vi "IMAQ FPGA Wait for Image Transfer Complete U8.vi"(5 "Wait Timeout (ms)":i32=5000, 7 "DMA FIFO Depth in Elements":u32, 8 "error in (no error)":errorcluster, 9 "DMA FIFO Reference In":refnum<k20>, 10 "Source FIFO Status Indicator Name":string, 11 "FPGA VI Reference In":refnum<k20>) -> (0 "error out":errorcluster, 1 "DMA FIFO Reference Out":refnum<k20>)   [LabVIEW 2020, in "NI_VDM_FPGA_Basics.lvlib"]
doc: "Waits for the transfer of image data from the host processor to the target FPGA via a DMA FIFO to complete or for the specified timeout to expire before returning. The transfer is deemed complete when the host-side buffer of the DMA FIFO is empty and the DMA FIFO on the FPGA is empty as well. To ensure that none of the image data will be lost, call this VI after the last call to the IMAQ FPGA Image Transfer to Target VI and prior to calling the Close FPGA VI Reference function on the DMA FIFO Reference."
uses:
  <vilib>/visionFPGA/NI_VDM_FPGA_Basics.lvlib
  <vilib>/visionFPGA/Controls/IMAQ FPGA Source FIFO Status.ctl
  <vilib>/NI/LVFPGA Adv Session Resources/OpenByNameSubVI.vi
  <vilib>/rvi/errors/niLvFpgaAdjustHostInterfaceError.vi
  <vilib>/rvi/interface/common/dynamic/niFpgaEscapeDelimiterAndNull.vi
  <vilib>/FPGAPlugInAG/Dynamic/niLvFpga_Close_Dynamic.vi
  <vilib>/rvi/interface/nirviMethod/nirviMethod.xnode
  <vilib>/NI/LVFPGA Adv Session Resources/OpenByName.xnode
  <vilib>/rvi/interface/nirviReadWriteControl/nirviReadWriteControl.xnode
  <vilib>/rvi/interface/nirviCloseFPGA/nirviCloseFPGA.xnode
  <vilib>/NI/LVFPGA Adv Session Resources/LVFPGAAdvSessionResources.lvlib
  NiFpgaLv.dll
  <vilib>/rvi/interface/Simulation/niFpgaSimulationCallBeginRW.vi
  <vilib>/FPGAPlugInAG/Dynamic/niLvFpga_WriteFifo_Dynamic.vi
  <vilib>/rvi/errors/niLvFpgaMergeErrorWithErrorCode.vi
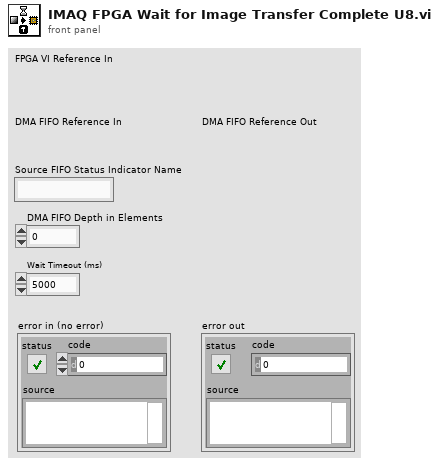
[diagram p1: front panel]
types:
  T1 = typedef "IMAQ FPGA Source FIFO Status.ctl" = cluster{"Number of Elements to Read":u32}
  T2 = enum16{"Register", "Host To Target FIFO", "Target To Host FIFO"}
  T3 = cluster{"Name":string, "Depth":u32, "Write? (Deprecated:Use Implementation)":bool, "Physical Channel":u32, "Base Address":u32, "Data Width":u32, "Data Type":enum32{"Boolean", "I8", "I16", "I32", "I64", "U8", "U16", "U32", "U64", "FXP", "CustomControl", "SGL"}, "FXP Properties":variant, "Write Window Address":u32, "Implementation":enum16{"niFpgaTargetToHost", "niFpgaHostToTarget", "niFpgaPeerToPeerWriter", "niFpgaPeerToPeerReader", "niCoreTargetToHost", "niCoreHostToTarget"}, "Control Set":u32}[]
  T4 = cluster{"Name":string, "type":variant, "indicator?":bool}[]
  T5 = typedef "LVFPGAAdvSessionResources.lvlib/ResourceInfo.ctl" = cluster{"Resource name":string, "Data type":variant, "Resource type":enum16{"Register", "Host To Target FIFO", "Target To Host FIFO"}}
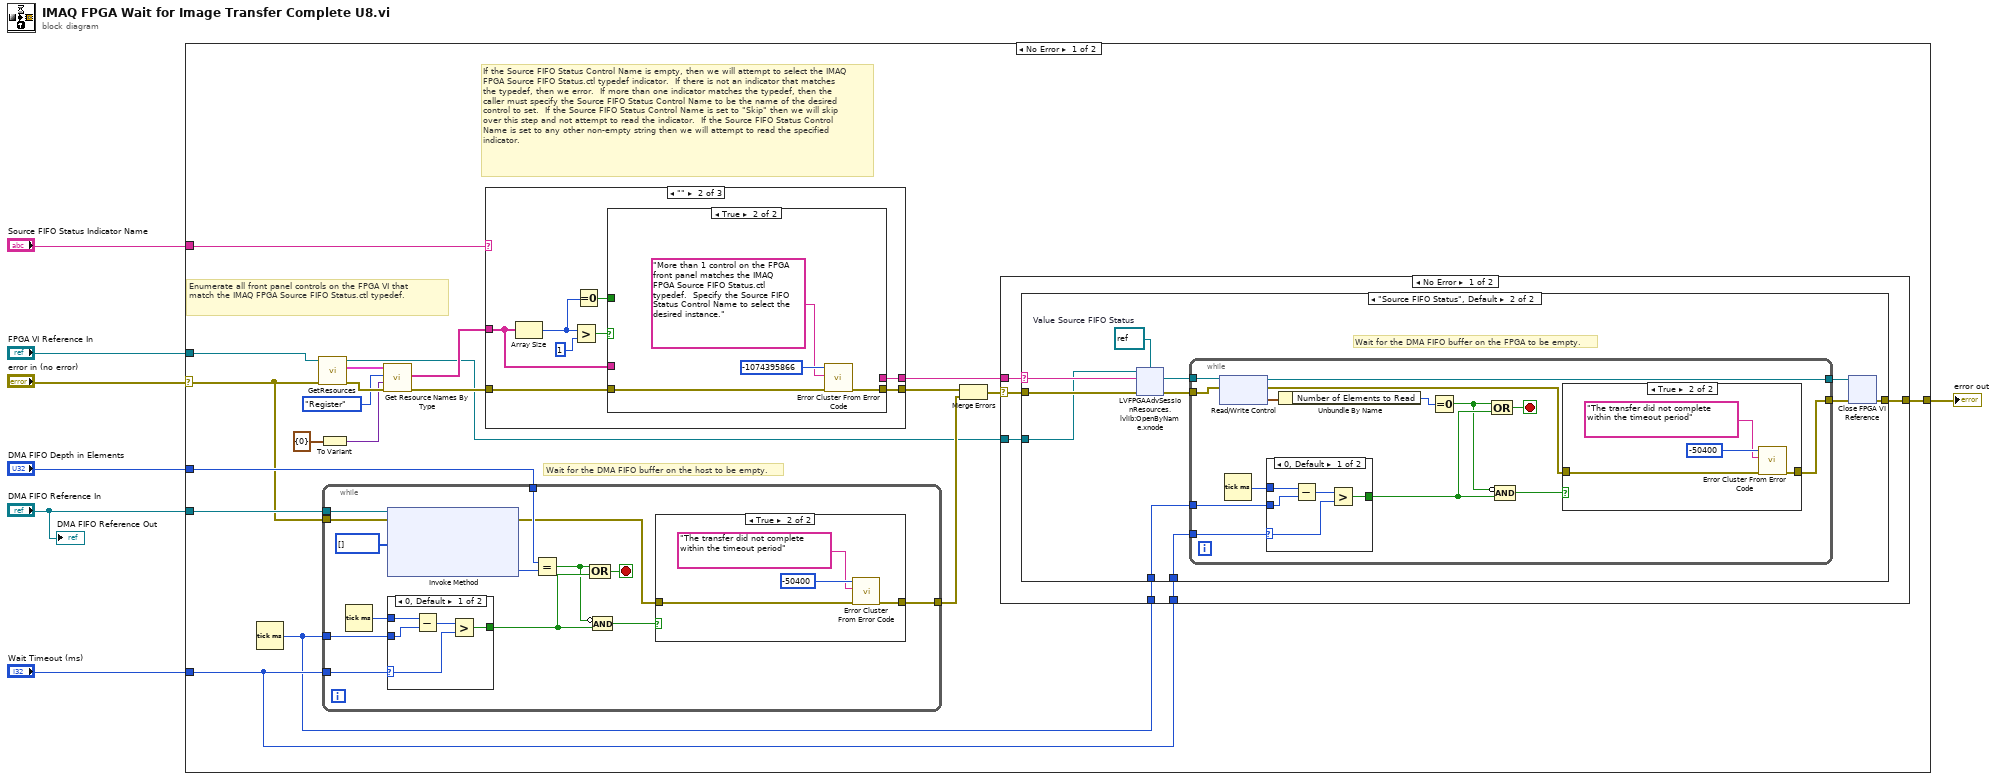
[diagram p0: block diagram]
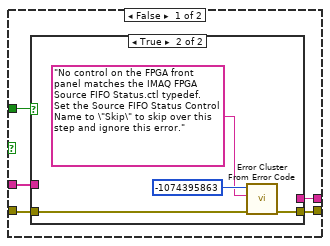
[diagram p7: hidden frame]
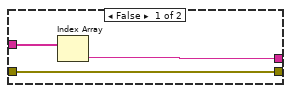
[diagram p8: hidden frame]
diagram:
  n1 = case shown="No Error" "error in (no error)" {
    selector: "error in (no error)" -> [w8 w135]
    tunnel: "DMA FIFO Depth in Elements" -> [w27 _]
    tunnel: "FPGA VI Reference In" -> [w23 _]
    tunnel: "Source FIFO Status Indicator Name" -> [w21 _]
    tunnel: "Wait Timeout (ms)" -> [w13 _]
    tunnel: [w11 w135] -> w3
    tunnel: "DMA FIFO Reference In" -> [w10 _]
    frame No Error {
      # "Wait for the DMA FIFO buffer on the host to be empty."
      # "If the Source FIFO Status Control Name is empty, then we will attempt to select the IMAQ FPGA Source FIFO Status.ctl typedef indicator.  If there is not an indicator that matches the typedef, then we error.  If more than one indicator matches the typedef, then the caller must specify the Source FIFO Status Control Name to be the name of the desired control to set.  If the Source FIFO Status Control Name is set to \"Skip\" then we will skip over this step and not attempt to read the indicator.  If the Source FIFO Status Control Name is set to any other non-empty string then we will attempt to read the specified indicator."
      # "Enumerate all front panel controls on the FPGA VI that match the IMAQ FPGA Source FIFO Status.ctl typedef."
      n2 = Tick Count (ms)() -> (millisecond timer value=w12:u32)
      n3 = call <vilib>:"GetResources.vi"("error in (no error)"=w8, "FPGA VI Reference in"=w23) -> ("error out"=w26:errorcluster, "Resource info out"=w24:T5[], "FPGA VI Reference out"=w14:refnum<k20>)  [unwired: 7 in]
      n4 = To Variant(anything=T1 {"Number of Elements to Read"=0} ("Source FIFO Status")) -> (Variant=w19:variant)
      n5 = while {
        tunnel: w10 -> [w124]
        tunnel: w27 -> [w122]
        tunnel: w8 -> [w121]
        tunnel: w12 -> [w118]
        tunnel: w13 -> [w119]
        tunnel: [w111] -> w16
        stop <- w116 stop-if-true
        n6 = Tick Count (ms)() -> (millisecond timer value=w117:u32)
        n7 = case shown="0, Default" w119 {
          selector: w119 -> [w131 _]
          tunnel: w118 -> [w133 _]
          tunnel: w117 -> [w134 _]
          tunnel: [w130 _] -> w115
          frame 0, Default {
            n8 = Subtract(x=w134, y=w133) -> (x-y=w132:u32)
            n9 = Greater?(x=w132, y=w131) -> (0:w130:bool)
          }
          frame -1 {
          }
        }
        n10 = xnode "Invoke Method"("FPGA VI Reference In"=w124, "error in"=w121, "Data"=u8[] []) -> ("error out"=w112:errorcluster, "Empty Elements Remaining"=w123:u32)  [unwired: 1 in, 1 out]
        n11 = Equal?(x=w122, y=w123) -> (x = y?=w114:bool)
        n12 = Compound Arithmetic op=OR(w114, w115) -> (w116:bool)
        n13 = Compound Arithmetic op=AND(invert w114, w115) -> (w113:bool)
        n14 = case shown="True" w113 {
          tunnel: w112 -> [w125 w129]
          tunnel: [w125 w128] -> w111
          frame False {
          }
          frame True {
            n15 = call <vilib>:"Error Cluster From Error Code.vi"("error in (no error)"=w129, "error message (\"\")"="The transfer did not complete within the timeout period" ("error message (\"\")"), "error code (0)"=-50400) -> ("error out"=w128:errorcluster)  [unwired: 6 in]
          }
        }
      }
      n16 = call <vilib>:"Get Resource Names By Type.vi"("error in (no error)"=w26, "Data Type"=w19, "Resource Type"=T2."Register", "Resource Info In"=w24) -> ("error out"=w20:errorcluster, "Resource Names"=w22:string[])  [unwired: 5 in, 1 out]
      n17 = case shown="\"\"" w21 {
        selector: w21 -> [w84 _ _]
        tunnel: w20 -> [w85 w92 w110]
        tunnel: [w85 w91 w110] -> w17
        tunnel: [w84 w90 _] -> w18
        tunnel: w22 -> [_ w88 _]
        frame "Anything Else", Default {
        }
        frame "" {
          n18 = Array Size(array=w88) -> (size(s)=w86:i32)
          n19 = Greater?(x=w86, y=1 ("x")) -> (0:w93:bool)
          n20 = Equal To 0?(x=w86) -> (x = 0?=w87:bool)
          n21 = case shown="True" w93 {
            tunnel: w88 -> [w98 _]
            tunnel: [w97 _] -> w90
            tunnel: [w95 w107] -> w91
            tunnel: w92 -> [w96 w106]
            tunnel: w87 -> [w94 _]
            frame False {
              n22 = case shown="True" w94 {
                tunnel: w98 -> [w101 _]
                tunnel: [w100 _] -> w97
                tunnel: w96 -> [w99 w103]
                tunnel: [w99 w102] -> w95
                frame False {
                  n23 = Index Array(array=w101) -> (element=w100:string)  [unwired: 1 in]
                }
                frame True {
                  n24 = call <vilib>:"Error Cluster From Error Code.vi"("error in (no error)"=w103, "error message (\"\")"="No control on the FPGA front panel matches the IMAQ FPGA Source FIFO Status.ctl typedef.  Set the Source FIFO Status Control Name to \"Skip\" to skip over this step and ignore this error." ("error message (\"\")"), "error code (0)"=-1074395863) -> ("error out"=w102:errorcluster)  [unwired: 6 in]
                }
              }
            }
            frame True {
              n25 = call <vilib>:"Error Cluster From Error Code.vi"("error in (no error)"=w106, "error message (\"\")"="More than 1 control on the FPGA front panel matches the IMAQ FPGA Source FIFO Status.ctl typedef.  Specify the Source FIFO Status Control Name to select the desired instance." ("error message (\"\")"), "error code (0)"=-1074395866) -> ("error out"=w107:errorcluster)  [unwired: 6 in]
            }
          }
        }
        frame "Skip" {
        }
      }
      n26 = Merge Errors(w17, w16) -> (w15:errorcluster)
      n27 = case shown="No Error" w15 {
        selector: w15 -> [w32 w83]
        tunnel: w18 -> [w33 _]
        tunnel: w14 -> [w31 _]
        tunnel: w13 -> [w30 _]
        tunnel: w12 -> [w29 _]
        tunnel: [w28 w83] -> w11
        frame No Error {
          n28 = case shown="\"Source FIFO Status\", Default" w33 {
            selector: w33 -> [_ w44]
            tunnel: w32 -> [w34 w43]
            tunnel: w31 -> [_ w42]
            tunnel: w30 -> [_ w37]
            tunnel: w29 -> [_ w36]
            tunnel: [w34 w35] -> w28
            frame "" {
            }
            frame "Source FIFO Status", Default {
              w45 = refnum<k20> refnum  # Value Source FIFO Status
              # "Wait for the DMA FIFO buffer on the FPGA to be empty."
              n29 = xnode "LVFPGAAdvSessionResources.lvlib:OpenByName.xnode"("FPGA VI Reference in"=w42, "Resource name in"=w44, "Single resource reference type in"=w45, "Error in"=w43) -> ("Single resource reference out"=w38:refnum<k20>, "Error out"=w41:errorcluster)  [unwired: 1 out]
              n30 = while {
                tunnel: w38 -> [w72]
                tunnel: w41 -> [w71]
                tunnel: [w59] -> w40
                tunnel: [w70] -> w39
                tunnel: w37 -> [w66]
                tunnel: w36 -> [w65]
                stop <- w64 stop-if-true
                n31 = xnode "Read/Write Control"("FPGA VI Reference In"=w72, "error in"=w71) -> ("FPGA VI Reference Out"=w70:refnum<k20>, "error out"=w61:errorcluster, "Value"=w68:cluster{"Number of Elements to Read":u32})
                n32 = Tick Count (ms)() -> (millisecond timer value=w67:u32)
                n33 = case shown="0, Default" w66 {
                  selector: w66 -> [w79 _]
                  tunnel: w65 -> [w81 _]
                  tunnel: w67 -> [w82 _]
                  tunnel: [w78 _] -> w63
                  frame 0, Default {
                    n34 = Subtract(x=w82, y=w81) -> (x-y=w80:u32)
                    n35 = Greater?(x=w80, y=w79) -> (0:w78:bool)
                  }
                  frame -1 {
                  }
                }
                n36 = Unbundle By Name(w68) -> ("Number of Elements to Read"=w69:u32)
                n37 = Equal To 0?(x=w69) -> (x = 0?=w62:bool)
                n38 = Compound Arithmetic op=OR(w62, w63) -> (w64:bool)
                n39 = Compound Arithmetic op=AND(invert w62, w63) -> (w60:bool)
                n40 = case shown="True" w60 {
                  tunnel: w61 -> [w73 w77]
                  tunnel: [w73 w76] -> w59
                  frame False {
                  }
                  frame True {
                    n41 = call <vilib>:"Error Cluster From Error Code.vi"("error in (no error)"=w77, "error message (\"\")"="The transfer did not complete within the timeout period" ("error message (\"\")"), "error code (0)"=-50400) -> ("error out"=w76:errorcluster)  [unwired: 6 in]
                  }
                }
              }
              n42 = xnode "Close FPGA VI Reference"("FPGA VI Reference In"=w39, "error in"=w40) -> ("error out"=w35:errorcluster)
            }
          }
        }
        frame Error {
        }
      }
    }
    frame Error {
    }
  }
  "error out" <- w3
  "DMA FIFO Reference Out" <- "DMA FIFO Reference In"
